vi "populateBroadcastStepMotorFrame.vi"(8 "error in (no error)":errorcluster, 10 "FixedFrameBuilder in":refnum<class "FixedFrameBuilder.lvclass">, 11 "HardPointActuator in":refnum<class "HPILC.lvclass">) -> (0 "error out":errorcluster, 2 "FixedFrameBuilder out":refnum<class "FixedFrameBuilder.lvclass">, 3 "HardPointActuator out":refnum<class "HPILC.lvclass">)   [LabVIEW 2015, in "RTHPILC.lvlib" / "HPILC.lvclass"]
uses:
  HPILC.lvclass
  Common_RT_Modbus/FixedFrameBuilder/FixedFrameBuilder.lvclass
  Common_RT_ILC/ILC/ILC.lvclass/ILC.ctl
  HPILC.lvclass/HPILC.ctl
  Common_RT_ILC/ILC/ILC.lvclass
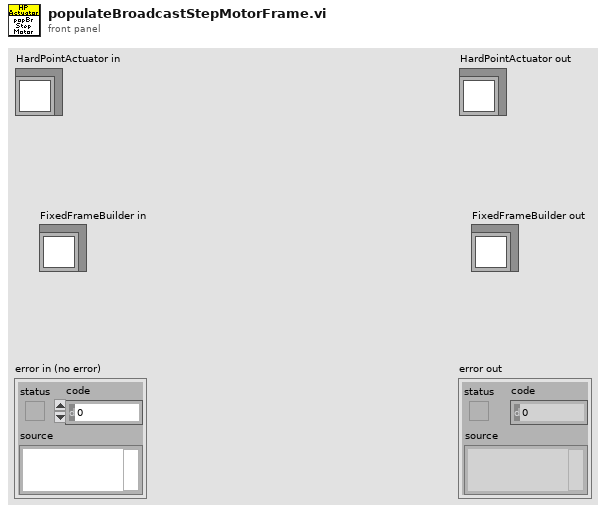
[diagram p1: front panel]
types:
  T1 = typedef "RTILC.lvlib/ILCData.ctl" = cluster{"Constants":T2, "Command":T3, "Telemetry":T4, "Responses":T5}
  T2 = typedef "RTILC.lvlib/ILCConstants.ctl" = cluster{"Subnet":u8, "Address":u8}
  T3 = typedef "RTILC.lvlib/ILCCommand.ctl" = cluster{"ILCMode":u16, "TemporaryAddress":u8}
  T4 = typedef "RTILC.lvlib/ILCTelemetry.ctl" = cluster{"UniqueID":u64, "FirmwareType":u8, "NetworkNodeType":u8, "ILCOption":u8, "NetworkNodeOption":u8, "MajorRevision":u8, "MinorRevision":u8, "FirmwareName":string, "ILCMode":u16, "MajorFault":bool, "MinorFault":bool, "FaultOverride":bool, "UniqueIDCRCMismatch":bool, "AppTypeNodeTypeMismatch":bool, "AppMissing":bool, "AppCRCMismatch":bool, "TEDSNotFound":bool, "TEDS1Mismatch":bool, "TEDS2Mismatch":bool, "WatchdogResetDetected":bool, "BrownoutDetected":bool, "EventTrapResetDetected":bool, "TemporaryAddress":u8}
  T5 = typedef "RTILC.lvlib/ILCResponses.ctl" = cluster{"ReportServerID":T6, "ReportServerStatus":T6, "ILCMode":T6, "SetTemporaryAddress":T6, "Reset":T6}
  T6 = typedef "RTModbus.lvlib/ExceptionCodes.ctl" = enum16{"None", "IllegalFunction", "IllegalDataAddress", "IllegalDataValue", "SlaveDeviceFailure", "Acknowledge", "SlaveDeviceBusy", "NegativeAcknowledge", "MemoryParityError", "GatewayPathUnavailable", "GatewayTargetDeviceFailedToRespond"}
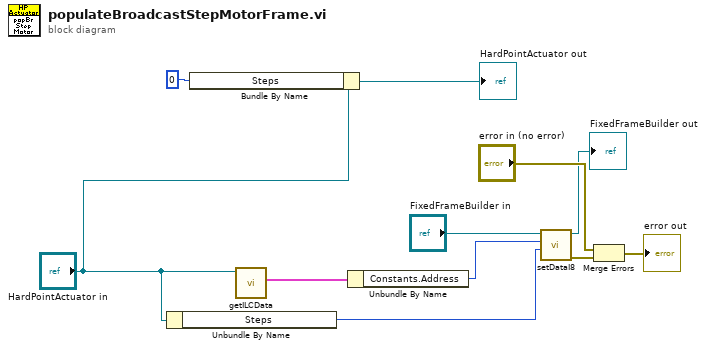
[diagram p0: block diagram]
diagram:
  n1 = Unbundle By Name("HardPointActuator in") -> ("Steps"=w7:i8)
  n2 = Bundle By Name(cluster="HardPointActuator in", "Steps"=i8 0 ("HPData.HPCommand.Steps")) -> (→"HardPointActuator out":refnum<class "HPILC.lvclass">)
  n3 = call "getILCData.vi"("ILC in"="HardPointActuator in") -> ("ILCData"=w9:T1)  [unwired: 9 in, 1 out]
  n4 = Unbundle By Name(w9) -> ("Constants.Address"=w1:u8)
  n5 = call "setDataI8.vi"("Data"=w7, "Index"=w1, "FixedFrameBuilder in"="FixedFrameBuilder in") -> ("error out"=w2:errorcluster, "FixedFrameBuilder out"=→"FixedFrameBuilder out":refnum<class "FixedFrameBuilder.lvclass">)  [unwired: 7 in]
  n6 = Merge Errors("error in (no error)", w2) -> (→"error out":errorcluster)
